vi "Kinesis - KDC101 - Move Absolute.vi"() -> ()   [LabVIEW 2024]
doc: "Shows how to move a motor to an absolute position."
uses:
  C:/Users/goods/OneDrive/Desktop/Work/program/MOVER/ThorLabs.MotionControl.KCube.DCServoCLI.dll
  ThorLabs.MotionControl.KCube.DCServoCLI.dll
  C:/Users/goods/OneDrive/Desktop/Work/program/MOVER/Thorlabs.MotionControl.Controls.dll
  Thorlabs.MotionControl.Controls.dll
panel:
  out "Waveform Chart":dbl(graph)
  out "Positon":string
  in  "SerialNumber":string
  in  "Abs Pos":dbl
  in  "Home":bool
  in  "MoveAbsolute":bool
  in  "Set Abs Pos":bool
  in  "?":bool
  in  "KCubeDCServoControl":refnum<k24>(container)
  # "Notes:"
  # "- Ensure that the appropriate .DLLs are copied into your Project Folder. Check that the correct bit type are used depending on your version of LabVIEW\ni.e. 32-bit or 64-bit.\n\n\n\n\n\n\n\n\n\n\n\n\n\n\n- Open the example VI through the LabVIEW Project Explorer to correctly load the User Interface from Thorlabs.MotionControl.Controls.dll."
  # "Thorlabs Hardware: KDC101 - K-Cube Brushless DC Servo Motor Controller\nhttps://www.thorlabs.com/thorproduct.cfm?partnumber=KDC101\n\nDescription: This VI will enable you to communicate with KDC101 to control DC Brushed Stages & Actuators. The VI will allow you to home the   device, and move it to any position without having to use the UI.\n\nInstructions: \n1) Connect your KDC101 device to your PC & power the device, ensuring your stage/actutator is connected. For full device setup, the device product manual can be found on our website here. - https://www.thorlabs.com/thorproduct.cfm?partnumber=KDC101\n2) Enter the device serial number below.\n3) Click 'Run' in the LabVIEW Toolbar.\n4) To end the Program click 'STOP'"
  # "Example Image of .NET Controller - VI opened via Project Explorer/ not opened via Project Explorer"
  # "VI Not Opened via Project Explorer"
  # "VI Opened via Project Explorer"
  # "- To explore the range of methods available, please visit the .NET API, included with your Kinesis software.\n\n- For tips on building your own VIs with Thorlabs Motion Control Hardware, please see our LabVIEW Guide here.\nhttps://www.thorlabs.com/newgrouppage9.cfm?objectgroup_id=10285"
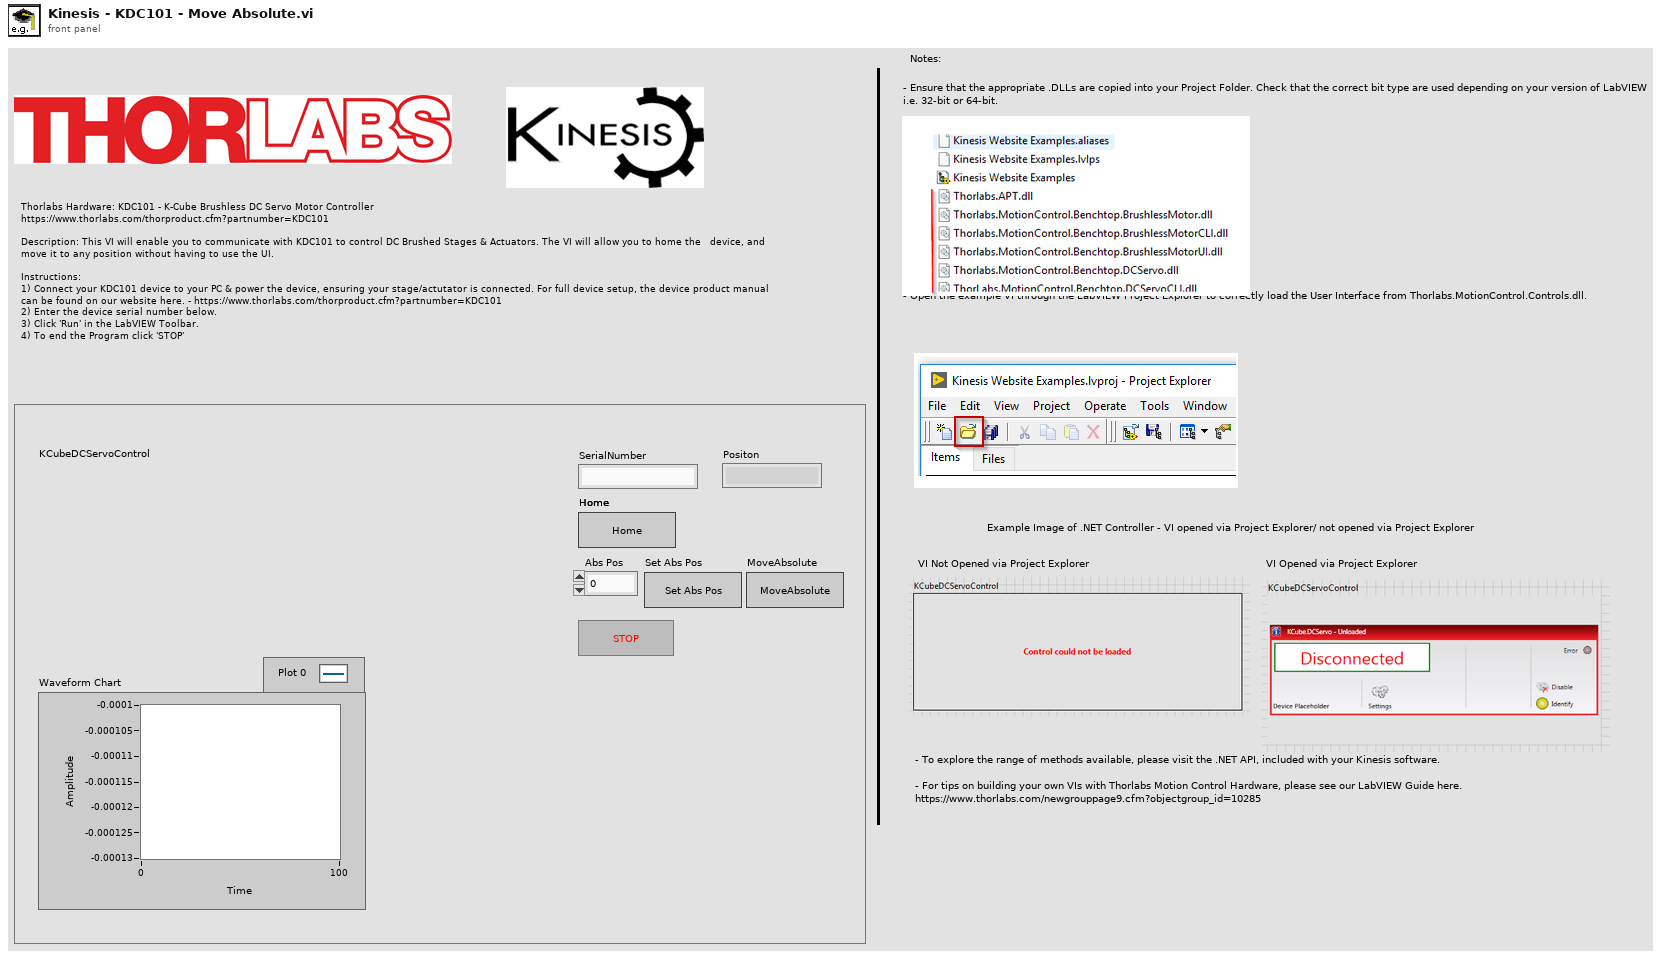
[diagram p1: front panel]
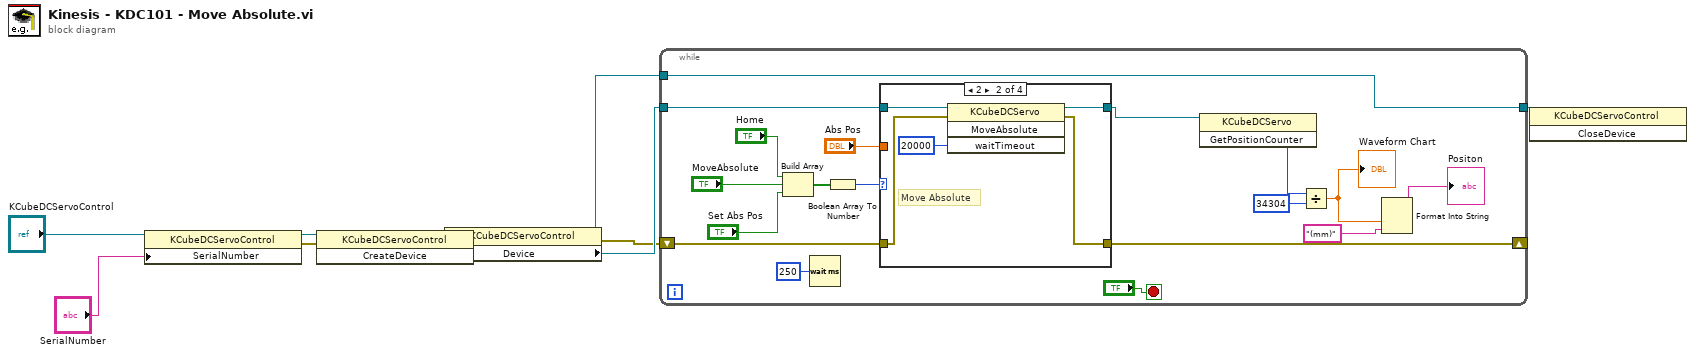
[diagram p0: block diagram]
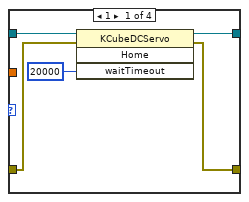
[diagram p2: hidden frame]
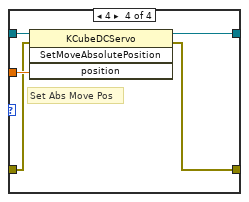
[diagram p4: hidden frame]
diagram:
  n1 = property class="KCubeDCServoControl"(reference="KCubeDCServoControl", "SerialNumber"="SerialNumber") -> (reference out=w9:refnum<k24>, error out=w6:errorcluster)  [unwired: 1 in]
  n2 = invoke class="KCubeDCServoControl" method="CreateDevice"(reference=w9, error in=w6) -> (reference out=w8:refnum<k24>, error out=w5:errorcluster)  [unwired: 1 in, 1 out]
  n3 = property class="KCubeDCServoControl"(reference=w8, error in=w5) -> (reference out=w2:refnum<k24>, error out=w4:errorcluster, "Device"=w7:refnum<k24>)
  n4 = while {
    tunnel: [w16] -> w1
    tunnel: w7 -> [w24]
    shift-right: [w21] -> _
    shift-left: w4 -> [w20]
    tunnel: w2 -> [w16]
    stop <- "?" stop-if-true
    n5 = Build Array("Home", "MoveAbsolute", "Set Abs Pos") -> (w23:bool[])
    n6 = Wait (ms)(milliseconds to wait=u32 250) -> ()  [unwired: 1 out]
    n7 = Boolean Array To Number(Boolean array=w23) -> (number=w22:u32)
    n8 = case shown="2" w22 {
      tunnel: w24 -> [w33 w37 w39 w45]
      tunnel: [w30 w35 w40 w42] -> w21
      tunnel: w20 -> [w31 w36 w40 w43]
      tunnel: "Abs Pos" -> [_ _ _ w44]
      tunnel: [w29 w34 w39 w41] -> w17
      frame 1 {
        n9 = invoke class="KCubeDCServo" method="Home"(reference=w33, error in=w31, "waitTimeout"=20000) -> (reference out=w29:refnum<k24>, error out=w30:errorcluster)  [unwired: 1 in, 2 out]
      }
      frame 2 {
        # "Move Absolute"
        n10 = invoke class="KCubeDCServo" method="MoveAbsolute"(reference=w37, error in=w36, "waitTimeout"=20000) -> (reference out=w34:refnum<k24>, error out=w35:errorcluster)  [unwired: 1 in, 2 out]
      }
      frame Default {
      }
      frame 4 {
        # "Set Abs Move Pos"
        n11 = invoke class="KCubeDCServo" method="SetMoveAbsolutePosition"(reference=w45, error in=w43, "position"=w44) -> (reference out=w41:refnum<k24>, error out=w42:errorcluster)  [unwired: 1 in, 2 out]
      }
    }
    n12 = invoke class="KCubeDCServo" method="GetPositionCounter"(reference=w17) -> ("GetPositionCounter"=w15:i32)  [unwired: 2 in, 2 out]
    n13 = Divide(x=w15, y=34304) -> (x/y=w11:dbl)
    "Waveform Chart" <- w11
    n14 = Format Into String(w11, "(mm)") -> (resulting string=→"Positon":string)  [unwired: 3 in, 1 out]
  }
  n15 = invoke class="KCubeDCServoControl" method="CloseDevice"(reference=w1) -> ()  [unwired: 2 in, 3 out]
